vi "Create Enumerator.vi"(8 "error in (no error)":errorcluster caption="错误输入（无错误）", 10 "Enumerator":refnum<k24>, 11 "Enumerator 输入":refnum<class "Enumerator.lvclass"> caption="DNL_LabVIEW Object in") -> (0 "error out":errorcluster caption="错误输出", 3 "Enumerator 输出":refnum<class "Enumerator.lvclass"> caption="DNL_LabVIEW Object out")   [LabVIEW 2012, in "Enumerator.lvclass"]
uses:
  Enumerator.lvclass
  Enumerator.lvclass/Enumerator.ctl
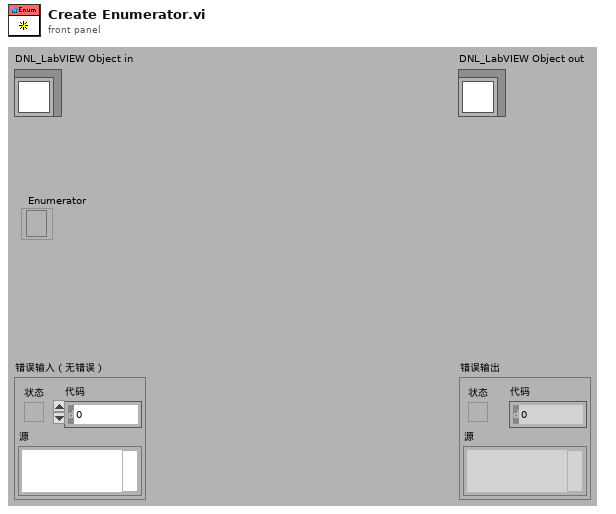
[diagram p1: front panel]
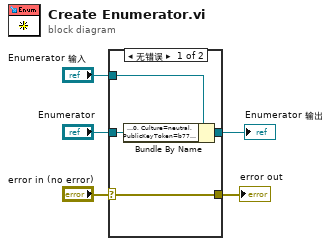
[diagram p0: block diagram]
diagram:
  n1 = case shown="无错误" "error in (no error)" {
    selector: "error in (no error)" -> [w9 w11]
    tunnel: [w9 w11] -> w4
    tunnel: [w7 w10] -> w2
    tunnel: "Enumerator 输入" -> [w8 w10]
    tunnel: "Enumerator" -> [w6 _]
    frame No Error {
      n2 = Bundle By Name(cluster=w8, "Enumerator"=w6) -> (w7:refnum<class "Enumerator.lvclass">)
    }
    frame Error {
    }
  }
  "error out" <- w4
  "Enumerator 输出" <- w2
